vi "My OFDM TX.vi"() -> ()   [LabVIEW 2013]
uses:
  <vilib>/Analysis/2dsp.llb/Inverse Complex FFT.vi
  <vilib>/addons/Modulation/Digital/General/MT Generate Bits (Galois, PN Order).vi
  <vilib>/addons/Modulation/Digital/General/MT Map Bits to QAM Symbols.vi
  <vilib>/addons/Modulation/niDMT.lvlib
  <vilib>/Analysis/NI_AALPro.lvlib
  <vilib>/addons/Modulation/niAMT.lvlib
panel:
  in  "desired sample rate (Hz)":dbl=1.0 format="%.2f"
  in  "stop":bool
  out "error out":errorcluster
  out "Complex baseband":cluster{"t0":dbl, "dt":dbl, "Y":dbl[]}[](graph)
  out "Outgoing Constellation":cdb[](graph)
  out "output bit stream":i8[](array[numeric])
  in  "error in (no error)":errorcluster
  in  "Number of Bits":i32=128 caption="total bits (128)"
  in  "Queue size":i32
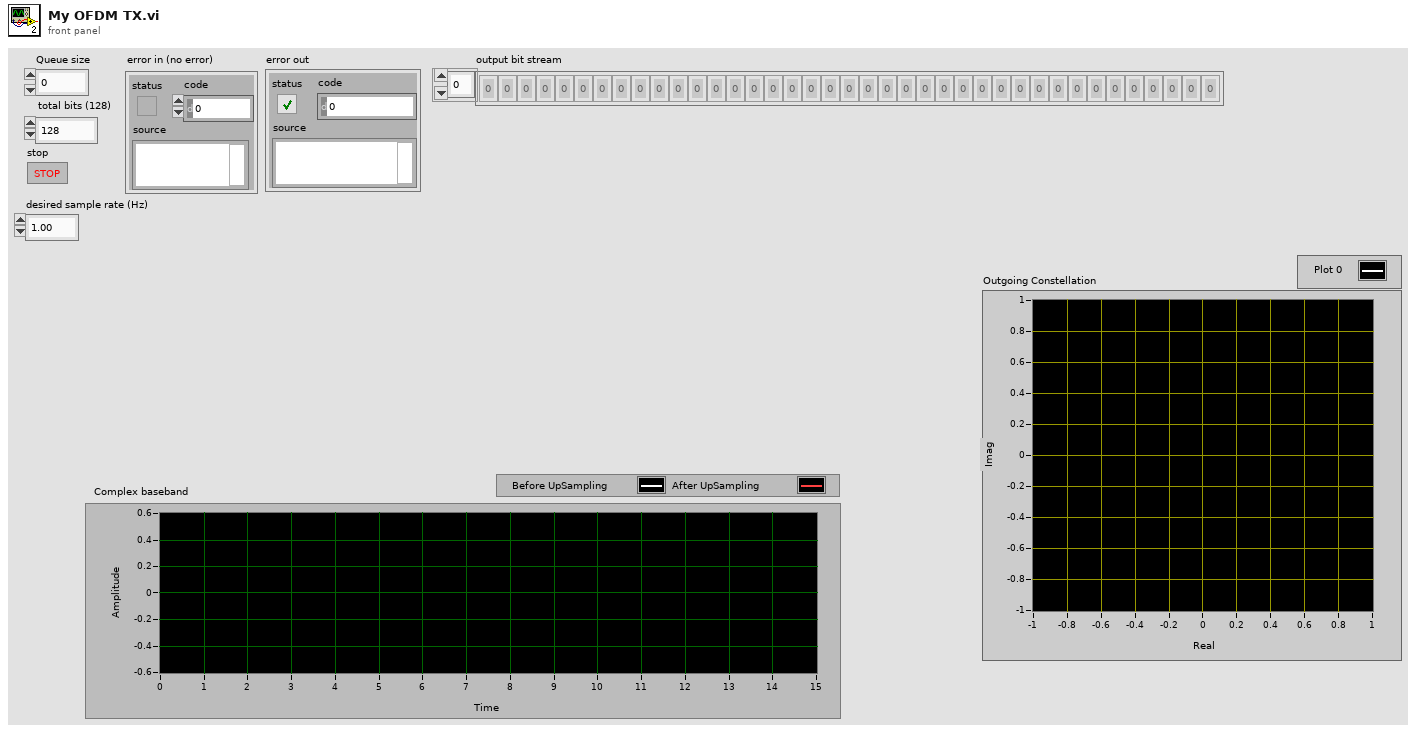
[diagram p1: front panel]
types:
  T1 = cluster{"IQ Data":cdb[], "Original Birstream":i8[]}
  T2 = typedef "niAMT.lvlib/Complex Data Waveform.ctl" = cluster{"t0":dbl, "dt":dbl, "Y":cdb[]}
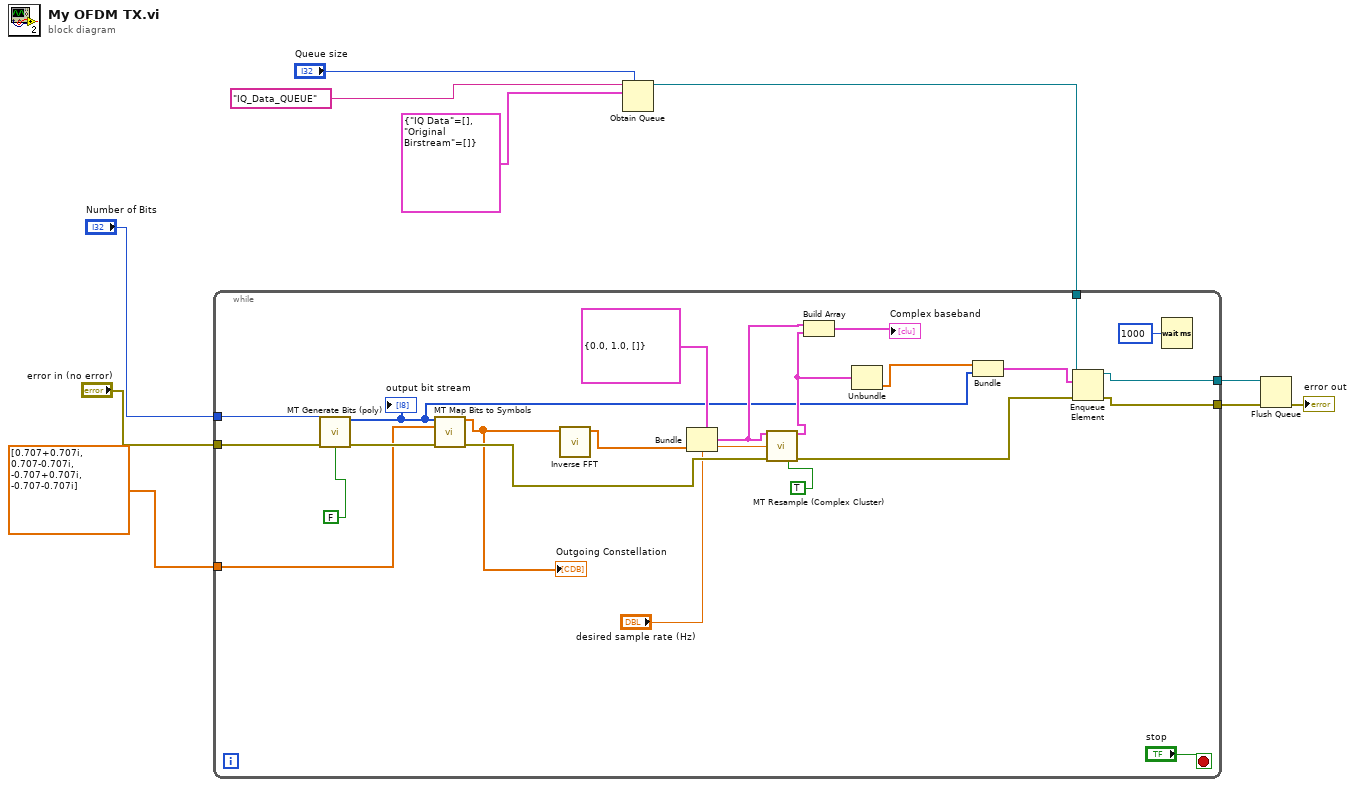
[diagram p0: block diagram]
diagram:
  n1 = Obtain Queue(max queue size (-1, unlimited)="Queue size", name (unnamed)="IQ_Data_QUEUE", element data type=T1 {"IQ Data"=[], "Original Birstream"=[]}) -> (queue out=w4:refnum<queue>)  [unwired: 2 in, 2 out]
  n2 = while {
    tunnel: "Number of Bits" -> [w33]
    tunnel: "error in (no error)" -> [w31]
    tunnel: cdb[] [0.707+0.707i, 0.707-0.707i, -0.707+0.707i, -0.707-0.707i] ("symbol map") -> [w29]
    tunnel: w4 -> [w17]
    tunnel: [w15] -> w3
    tunnel: [w14] -> w2
    stop <- "stop" stop-if-true
    n3 = call-poly <vilib>:"MT Generate Bits (poly).vi"("total bits (128)"=w33, "error in (no error)"=w31, "reset? (T)"=FALSE) -> ("output bit stream"=w19:i8[], "error out"=w30:errorcluster)  [unwired: 10 in, 1 out]
    "output bit stream" <- w19
    n4 = call-poly <vilib>:"MT Map Bits to Symbols.vi"("input bit stream"=w19, "symbol map"=w29, "error in (no error)"=w30) -> ("symbols"=w22:cdb[], "error out"=w25:errorcluster)  [unwired: 11 in]
    "Outgoing Constellation" <- w22
    n5 = call-poly <vilib>:"Inverse FFT.vi"("FFT {X}"=w22) -> ("X"=w28:cdb[])  [unwired: 9 in, 1 out]
    n6 = Bundle(cluster=cluster{dbl, dbl, cdb[]} {0.0, 1.0, []}, w28) -> (w26:cluster{dbl, dbl, cdb[]})  [unwired: 2 in]
    n7 = call <vilib>:"MT Resample (Complex Cluster).vi"("input complex waveform"=w26, "desired sample rate (Hz)"="desired sample rate (Hz)", "error in (no error)"=w25, "flush buffers? (F)"=TRUE) -> ("output complex waveform"=w23:T2, "error out"=w16:errorcluster)  [unwired: 10 in]
    n8 = Build Array(w26, w23) -> (→"Complex baseband":T2[])
    n9 = Unbundle(w23) -> ("Y"=w20:cdb[])  [unwired: 2 out]
    n10 = Bundle("Y"=w20, "output bit stream"=w19) -> (w18:cluster{"Y":cdb[], "output bit stream":i8[]})  [unwired: 1 in]
    n11 = Enqueue Element(queue=w17, element=w18, error in (no error)=w16) -> (queue out=w15:refnum<queue>, error out=w14:errorcluster)  [unwired: 1 in, 1 out]
    n12 = Wait (ms)(milliseconds to wait=u32 1000) -> ()  [unwired: 1 out]
  }
  n13 = Flush Queue(queue=w3, error in (no error)=w2) -> (error out=→"error out":errorcluster)  [unwired: 2 out]
